vi "VI Hovacal.vi"(6 "Enum":T1, 8 "error in (no error)":errorcluster caption="Fehler (Eingang, kein Fehler)", 11 "VISA":refnum<visa-resource-name>="COM2") -> (0 "error out":errorcluster, 3 "Device":string)   [LabVIEW 2015, in "Linearisierung V2.lvlib" / "Gasteiler.lvlib" / "HovaCal.lvlib"]
uses:
  HovaCal.lvlib
  Aktion_FGV_Kom.ctl
  Gase.ctl
  Vaporizer.ctl
  Betriebsdaten.ctl
panel:
  out "Fehler Kommunikation\nGase":bool
  out "Fehler Kommunikaton\nBetriebsdaten":bool
  out "Fehler Kommunikation\nVaporizer":bool
  in  "Standartwerte 3":bool
  in  "Vaporizer":bool
  in  "Vaporizer 2":T2={"Pumpe Ein/Aus"=0.0, "Wasser / Reagent"=0.0, "Reagent dry / wet"=0.0, "Reagent"=4.0, "min. Temperatur\n160 °C"=160.0, "Solltemperatur"=180.0, "Wasserkonzentration\nSoll"=0.0} caption="Vaporizer" {"Reagent" items=["HCI", "HF", "NH3", "Hg", "ppm", "Organik"]; "Reagent dry / wet" items=["wet", "dry"]; "Wasser / Reagent" items=["Wasser", "Reagent"]; "Pumpe Ein/Aus" items=["AUS", "EIN"]}
  in  "Gase":T3 {"Komponente 2" items=["Konzentration<1%", "CO2-15%", "O2-20%", "NH3-1%", "NO-5000"]; "Komponente 1" items=["Konzentration<1%", "CO2-15%", "O2-20%", "NH3-1%", "NO-5000"]; "Trägergas" items=["N2/AIR", "Fehler"]}
  in  "Daten":T4={"Gesamtdurchfluss"=3.0, "Eingangskonzentration \nTrägergas"=0.0, "Eingangskonzentration\nKomponente 1"=0.0, "Eingangskonzentration \nKomponente 2"=0.0, "Ausgangskonzentration \nKomponente 1 "=0.0, "Ausgangskonzentration\nKomponente 2"=0.0, "l/min -> ml/min"=FALSE, "N2 %->ppm"=FALSE, "Komp1 ppm->%"=FALSE, "Komp2ppm->%"=FALSE, "Sollkomp1ppm->%"=FALSE, "Sollkomp2ppm->%"=FALSE}
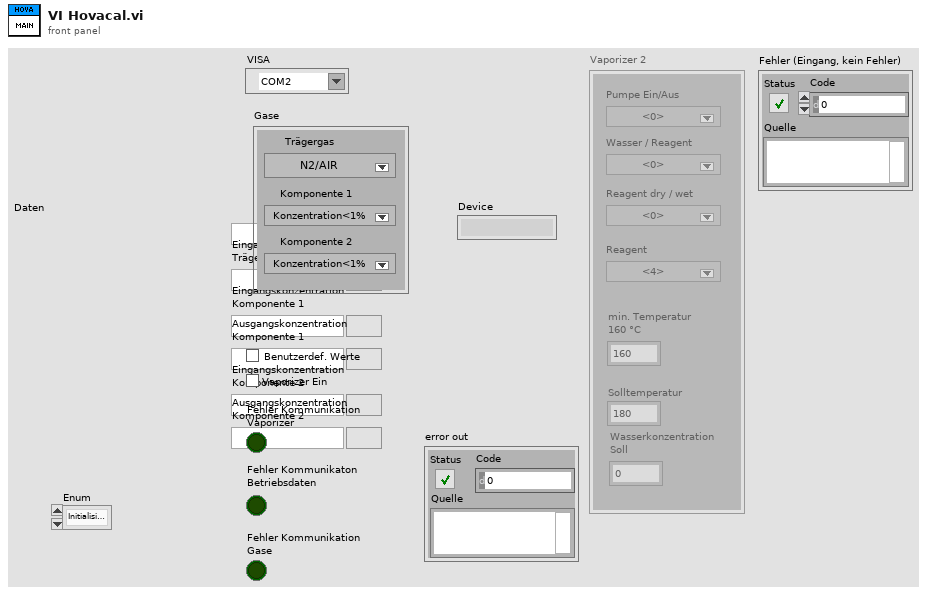
[diagram p1: front panel]
types:
  T1 = typedef "Linearisierung V2.lvlib/Gasteiler.lvlib/HovaCal.lvlib/Aktion_FGV_Kom.ctl" = enum16{"Initialisieren", "Betriebsparameter", "Gase", "Vaporizer", "Dynamische Werte", "Beenden", "Com ändern", "Gase init"}
  T2 = typedef "Linearisierung V2.lvlib/Gasteiler.lvlib/HovaCal.lvlib/Vaporizer.ctl" = cluster{"Pumpe Ein/Aus":dbl, "Wasser / Reagent":dbl, "Reagent dry / wet":dbl, "Reagent":dbl, "min. Temperatur\n160 °C":dbl, "Solltemperatur":dbl, "Wasserkonzentration\nSoll":dbl}
  T3 = typedef "Linearisierung V2.lvlib/Gasteiler.lvlib/HovaCal.lvlib/Gase.ctl" = cluster{"Trägergas":u16, "Komponente 1":u16, "Komponente 2":u16}
  T4 = typedef "Linearisierung V2.lvlib/Gasteiler.lvlib/HovaCal.lvlib/Betriebsdaten.ctl" = cluster{"Gesamtdurchfluss":dbl, "Eingangskonzentration \nTrägergas":dbl, "Eingangskonzentration\nKomponente 1":dbl, "Eingangskonzentration \nKomponente 2":dbl, "Ausgangskonzentration \nKomponente 1 ":dbl, "Ausgangskonzentration\nKomponente 2":dbl, "l/min -> ml/min":bool, "N2 %->ppm":bool, "Komp1 ppm->%":bool, "Komp2ppm->%":bool, "Sollkomp1ppm->%":bool, "Sollkomp2ppm->%":bool}
  T5 = enum16{"Lesen", "Sollwerte schreiben", "Sollwerte lesen", "Gase schreiben", "Gase lesen", "Dynamische Werte"}
  T6 = enum16{"Lesen", "Vaporizer lesen", "Vaporizer schreiben"}
  T7 = enum8{"Enabled", "Disabled", "Disabled and Grayed Out"}
  T8 = cluster{"Gesamtdurchfluss":bool, "Eingangskonzentration \nTrägergas":bool, "Eingangskonzentration\nKomponente 1":bool, "Eingangskonzentration \nKomponente 2":bool, "Ausgangskonzentration \nKomponente 1 ":bool, "Ausgangskonzentration\nKomponente 2":bool, "l/min -> ml/min":bool, "N2 %->ppm":bool, "Komp1 ppm->%":bool, "Komp2ppm->%":bool, "Sollkomp1ppm->%":bool, "Sollkomp2ppm->%":bool}
  T9 = cluster{"Pumpe Ein/Aus":bool, "Wasser / Reagent":bool, "Reagent dry / wet":bool, "Reagent":bool, "min. Temperatur\n160 °C":bool, "Solltemperatur":bool, "Wasserkonzentration\nSoll":bool}
  T10 = cluster{"Trägergas":bool, "Komponente 1":bool, "Komponente 2":bool}
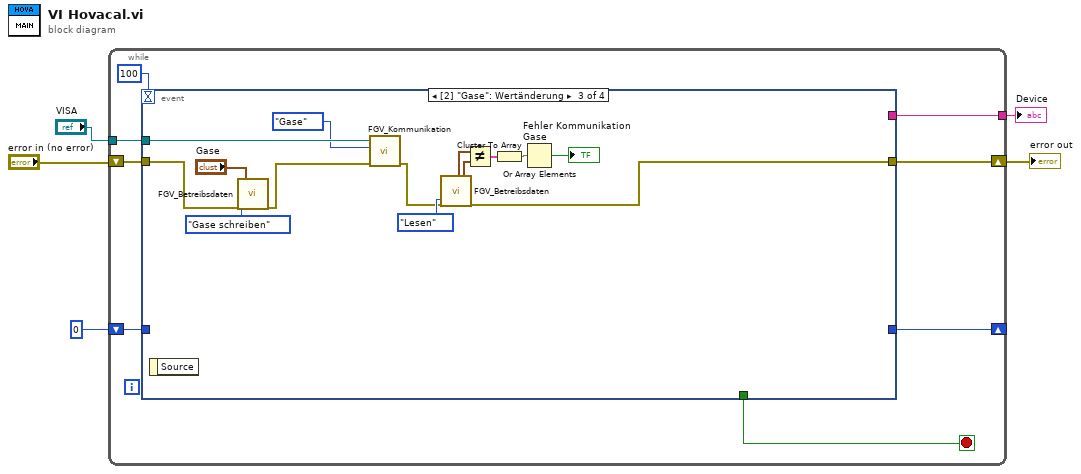
[diagram p0: block diagram]
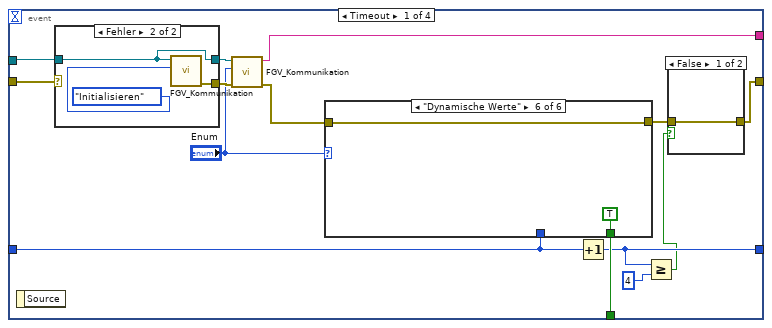
[diagram p2: hidden frame]
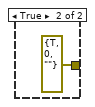
[diagram p4: hidden frame]
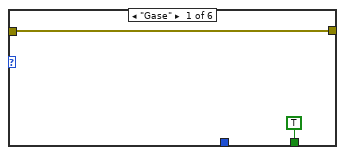
[diagram p5: hidden frame]
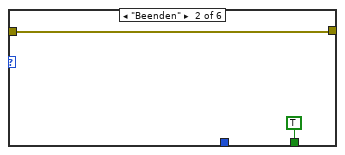
[diagram p6: hidden frame]
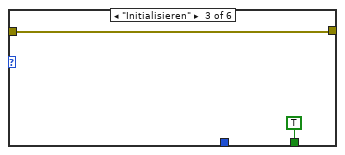
[diagram p7: hidden frame]
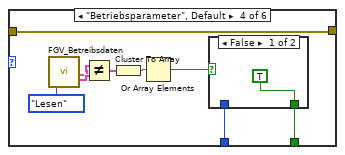
[diagram p8: hidden frame]
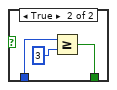
[diagram p9: hidden frame]
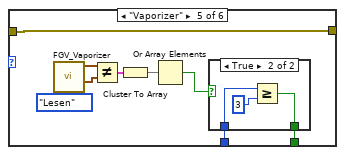
[diagram p10: hidden frame]
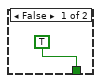
[diagram p11: hidden frame]
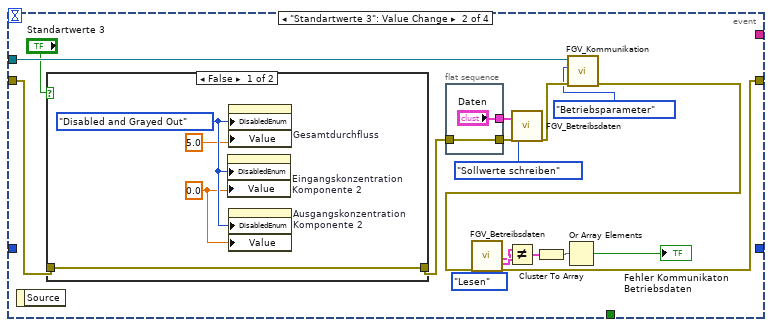
[diagram p12: hidden frame]
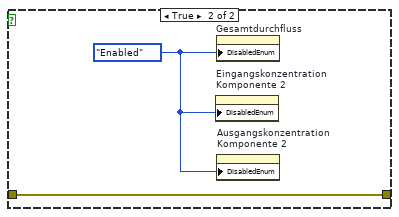
[diagram p13: hidden frame]
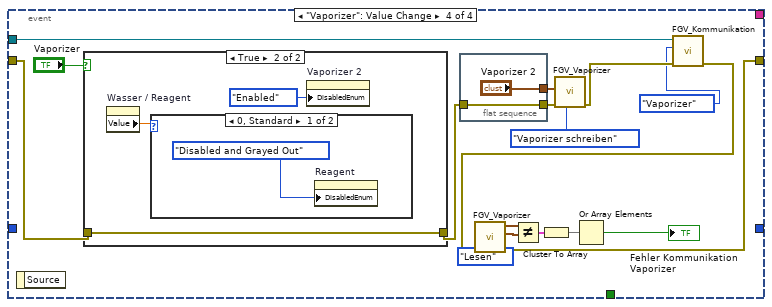
[diagram p14: hidden frame]
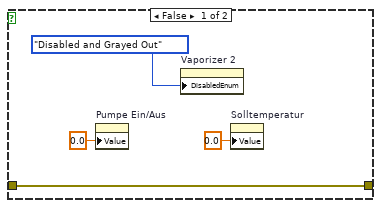
[diagram p15: hidden frame]
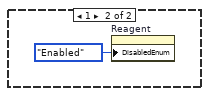
[diagram p16: hidden frame]
diagram:
  n1 = while {
    tunnel: "VISA" -> [w13]
    shift-right: [w12] -> w3
    shift-left: "error in (no error)" -> [w11]
    shift-right: [w7] -> _
    shift-left: 0 -> [w8]
    tunnel: [w6] -> w1
    stop <- w9 stop-if-true
    n2 = event shown="[2] \"Gase\": Wertänderung" {
      selector: _ -> [_ _ _ _]
      dyn-events: _ -> [_ _ _ _]
      timeout: 100 -> [_ _ _ _]
      tunnel: w13 -> [w26 w85 w107 w124]
      tunnel: [w19 w73 w95 w112] -> w12
      tunnel: w11 -> [w17 w80 w104 w122]
      tunnel: [w25 _ _ _] -> w9
      tunnel: w8 -> [w23 _ _ _]
      tunnel: [w22 _ _ _] -> w7
      tunnel: [w15 _ _ _] -> w6
      event Timeout {
        n3 = event-data() -> ()  [unwired: 1 in, 1 out]
        n4 = case shown="Fehler" w17 {
          selector: w17 -> [w29 _]
          tunnel: [w29 w32] -> w27
          tunnel: w26 -> [w28 w31]
          tunnel: [w28 w31] -> w16
          frame No Error {
          }
          frame Error {
            n5 = call "FGV_Kommunikation.vi"("Aktion"=Aktion_FGV_Kom."Initialisieren" ("Enum"), "VISA"=w31) -> ("error out"=w32:errorcluster)  [unwired: 7 in, 2 out]
          }
        }
        n6 = call "FGV_Kommunikation.vi"("error in"=w27, "Aktion"="Enum", "VISA"=w16) -> ("error out"=w24:errorcluster, "Device"=w15:string)  [unwired: 6 in, 1 out]
        n7 = case shown="\"Dynamische Werte\"" "Enum" {
          tunnel: [TRUE TRUE TRUE w44 w55 TRUE] -> w25
          tunnel: w24 -> [w36 w38 w40 w42 w58 w68]
          tunnel: [w36 w38 w40 w42 w58 w68] -> w18
          tunnel: w23 -> [_ _ _ w41 w56 _]
          frame "Gase" {
          }
          frame "Beenden" {
          }
          frame "Initialisieren" {
          }
          frame "Betriebsparameter", Default {
            n8 = call "FGV_Betreibsdaten.vi"(7:T5."Lesen" ("Enum")) -> ("Sollwerte lesen"=w45:T4, "Sollwert für Vergleich"=w46:T4)  [unwired: 11 in, 6 out]
            n9 = Not Equal?(x=w45, y=w46) -> (x != y?=w49:T8)
            n10 = Cluster To Array(cluster=w49) -> (array=w48:bool[])
            n11 = Or Array Elements(Boolean array=w48) -> (logical OR=w43:bool)
            n12 = case shown="False" w43 {
              tunnel: [TRUE w53] -> w44
              tunnel: w41 -> [_ w52]
              frame False {
              }
              frame True {
                n13 = Greater Or Equal?(x=w52, y=3) -> (x >= y?=w53:bool)
              }
            }
          }
          frame "Vaporizer" {
            n14 = call "FGV_Vaporizer.vi"("Enum"=T6."Lesen") -> ("Vaporizer %"=w54:T2, "Vaporizer_lesen"=w61:T2)  [unwired: 7 in, 2 out]
            n15 = Not Equal?(x=w61, y=w54) -> (x != y?=w60:T9)
            n16 = Cluster To Array(cluster=w60) -> (array=w59:bool[])
            n17 = Or Array Elements(Boolean array=w59) -> (logical OR=w57:bool)
            n18 = case shown="True" w57 {
              tunnel: [TRUE w64] -> w55
              tunnel: w56 -> [_ w66]
              frame False {
              }
              frame True {
                n19 = Greater Or Equal?(x=w66, y=3) -> (x >= y?=w64:bool)
              }
            }
          }
          frame "Dynamische Werte" {
          }
        }
        n20 = Increment(x=w23) -> (x+1=w22:i32)
        n21 = Greater Or Equal?(x=w22, y=4) -> (x >= y?=w20:bool)
        n22 = case shown="False" w20 {
          tunnel: [w33 errorcluster {"status"=TRUE, "code"=0, "source"=""} ("error out")] -> w19
          tunnel: w18 -> [w33 _]
          frame False {
          }
          frame True {
          }
        }
      }
      event "Standartwerte 3": Value Change {
        n23 = event-data() -> ()  [unwired: 1 in, 1 out]
        n24 = case shown="False" "Standartwerte 3" {
          tunnel: w80 -> [w90 w92]
          tunnel: [w90 w92] -> w79
          frame False {
            w88 = 0.0 ("Wert")
            w91 = T7."Disabled and Grayed Out" ("Deaktiviert")
            n25 = property on="Eingangskonzentration \nKomponente 2" class="DigWert (strikt)"("DisabledEnum"=w91, "Value"=w88) -> ()  [unwired: 2 in, 2 out]
            n26 = property on="Gesamtdurchfluss" class="DigWert (strikt)"("DisabledEnum"=w91, "Value"=5.0 ("Wert")) -> ()  [unwired: 2 in, 2 out]
            n27 = property on="Ausgangskonzentration\nKomponente 2" class="DigWert (strikt)"("DisabledEnum"=w91, "Value"=w88) -> ()  [unwired: 2 in, 2 out]
          }
          frame True {
            w93 = T7."Enabled" ("Deaktiviert")
            n28 = property on="Eingangskonzentration \nKomponente 2" class="DigWert (strikt)"("DisabledEnum"=w93) -> ()  [unwired: 2 in, 2 out]
            n29 = property on="Gesamtdurchfluss" class="DigWert (strikt)"("DisabledEnum"=w93) -> ()  [unwired: 2 in, 2 out]
            n30 = property on="Ausgangskonzentration\nKomponente 2" class="DigWert (strikt)"("DisabledEnum"=w93) -> ()  [unwired: 2 in, 2 out]
          }
        }
        n31 = flat-sequence {
          tunnel: ["Daten"] -> w83
          tunnel: w79 -> [w86]
          tunnel: [w86] -> w78
          frame #0 {
          }
        }
        n32 = call "FGV_Betreibsdaten.vi"("Sollwert schreiben"=w83, "error in (no error)"=w78, 7:T5."Sollwerte schreiben" ("Enum")) -> ("error out"=w82:errorcluster)  [unwired: 9 in, 7 out]
        n33 = call "FGV_Kommunikation.vi"("error in"=w82, "Aktion"=Aktion_FGV_Kom."Betriebsparameter" ("Enum"), "VISA"=w85) -> ("error out"=w74:errorcluster)  [unwired: 6 in, 2 out]
        n34 = call "FGV_Betreibsdaten.vi"("error in (no error)"=w74, 7:T5."Lesen" ("Enum")) -> ("Sollwerte lesen"=w70:T4, "Sollwert für Vergleich"=w71:T4, "error out"=w73:errorcluster)  [unwired: 10 in, 5 out]
        n35 = Not Equal?(x=w70, y=w71) -> (x != y?=w76:T8)
        n36 = Cluster To Array(cluster=w76) -> (array=w75:bool[])
        n37 = Or Array Elements(Boolean array=w75) -> (logical OR=→"Fehler Kommunikaton\nBetriebsdaten":bool)
      }
      event Value Change {
        n38 = event-data() -> ()  [unwired: 1 in, 1 out]
        n39 = call "FGV_Betreibsdaten.vi"("error in (no error)"=w104, "Gase schreiben"="Gase", 7:T5."Gase schreiben" ("Enum")) -> ("error out"=w103:errorcluster)  [unwired: 9 in, 7 out]
        n40 = call "FGV_Kommunikation.vi"("error in"=w103, "Aktion"=Aktion_FGV_Kom."Gase" ("Enum"), "VISA"=w107) -> ("error out"=w96:errorcluster)  [unwired: 6 in, 2 out]
        n41 = call "FGV_Betreibsdaten.vi"("error in (no error)"=w96, 7:T5."Lesen" ("Enum")) -> ("Gase schreiben"=w97:T3, "Gase lesen"=w98:T3, "error out"=w95:errorcluster)  [unwired: 10 in, 5 out]
        n42 = Not Equal?(x=w97, y=w98) -> (x != y?=w100:T10)
        n43 = Cluster To Array(cluster=w100) -> (array=w99:bool[])
        n44 = Or Array Elements(Boolean array=w99) -> (logical OR=→"Fehler Kommunikation\nGase":bool)
      }
      event "Vaporizer": Value Change {
        n45 = event-data() -> ()  [unwired: 1 in, 1 out]
        n46 = case shown="True" "Vaporizer" {
          tunnel: w122 -> [w127 w131]
          tunnel: [w127 w131] -> w120
          frame False {
            n47 = property on="Pumpe Ein/Aus" class="Ring (strikt)"("Value"=0.0 ("Wert")) -> ()  [unwired: 2 in, 2 out]
            n48 = property on="Vaporizer 2" class="Cluster (strikt)"("DisabledEnum"=T7."Disabled and Grayed Out" ("Deaktiviert")) -> ()  [unwired: 2 in, 2 out]
            n49 = property on="Solltemperatur" class="DigWert (strikt)"("Value"=0.0 ("Wert")) -> ()  [unwired: 2 in, 2 out]
          }
          frame True {
            n50 = property on="Wasser / Reagent" class="Ring (strikt)"() -> ("Value"=w132:dbl)  [unwired: 2 in, 2 out]
            n51 = case shown="0, Standard" w132 {
              frame 0, Default {
                n52 = property on="Reagent" class="Ring (strikt)"("DisabledEnum"=T7."Disabled and Grayed Out" ("Deaktiviert")) -> ()  [unwired: 2 in, 2 out]
              }
              frame 1 {
                n53 = property on="Reagent" class="Ring (strikt)"("DisabledEnum"=T7."Enabled" ("Deaktiviert")) -> ()  [unwired: 2 in, 2 out]
              }
            }
            n54 = property on="Vaporizer 2" class="Cluster (strikt)"("DisabledEnum"=T7."Enabled" ("Deaktiviert")) -> ()  [unwired: 2 in, 2 out]
          }
        }
        n55 = flat-sequence {
          tunnel: ["Vaporizer 2"] -> w111
          tunnel: [w125] -> w109
          tunnel: w120 -> [w125]
          frame #0 {
          }
        }
        n56 = call "FGV_Vaporizer.vi"("Enum"=T6."Vaporizer schreiben", "error in (no error)"=w109, "Vaporizer schreiben"=w111) -> ("error out"=w123:errorcluster)  [unwired: 5 in, 3 out]
        n57 = call "FGV_Kommunikation.vi"("error in"=w123, "Aktion"=Aktion_FGV_Kom."Vaporizer" ("Enum"), "VISA"=w124) -> ("error out"=w113:errorcluster)  [unwired: 6 in, 2 out]
        n58 = call "FGV_Vaporizer.vi"("Enum"=T6."Lesen", "error in (no error)"=w113) -> ("error out"=w112:errorcluster, "Vaporizer_schreiben"=w118:T2, "Vaporizer_lesen"=w117:T2)  [unwired: 6 in, 1 out]
        n59 = Not Equal?(x=w117, y=w118) -> (x != y?=w116:T9)
        n60 = Cluster To Array(cluster=w116) -> (array=w115:bool[])
        n61 = Or Array Elements(Boolean array=w115) -> (logical OR=→"Fehler Kommunikation\nVaporizer":bool)
      }
    }
  }
  "error out" <- w3
  "Device" <- w1
